vi "Set One Filter.vi"(8 "error in (no error)":errorcluster, 9 "Position (0:4)":i32, 10 "Filter Wheel (0:n-1)":i32, 11 "Filter Wheel in":refnum<class "Filter Wheel.lvclass">) -> (0 "error out":errorcluster, 1 "Target Counts":i32, 2 "Curr Pos":i32, 3 "Filter Wheel out":refnum<class "Filter Wheel.lvclass">, 4 "Message":string, 6 "No Move?":bool)   [LabVIEW 2024, in "Filter Wheel.lvclass"]
uses:
  Filter Wheel Object/Filter Wheel.lvclass
  Filter Wheel Object/Filter Wheel.lvclass/Filter Wheel.ctl
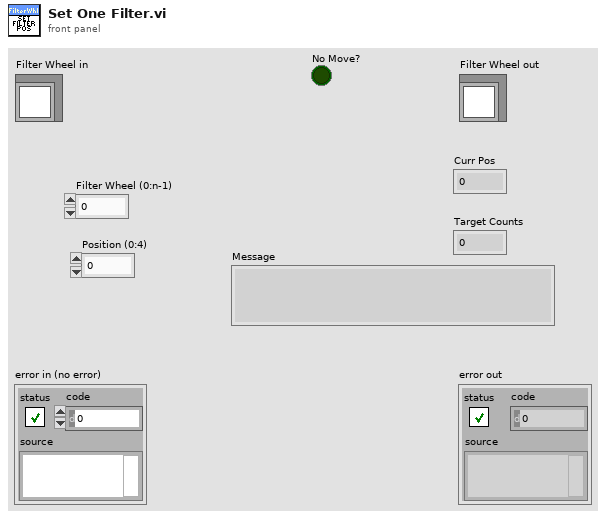
[diagram p1: front panel]
types:
  T1 = typedef "Filter Wheel Simulator.lvclass/Filter Wheel Move cluster.ctl" = cluster{"Wheel":i32, "Target Pos":i32}
  T2 = typedef "Filter Wheel.lvclass/Filter Wheel Details.ctl" = cluster{"Names":string[], "Relative Position":i32[], "Wheel Name":string, "Size":i32}
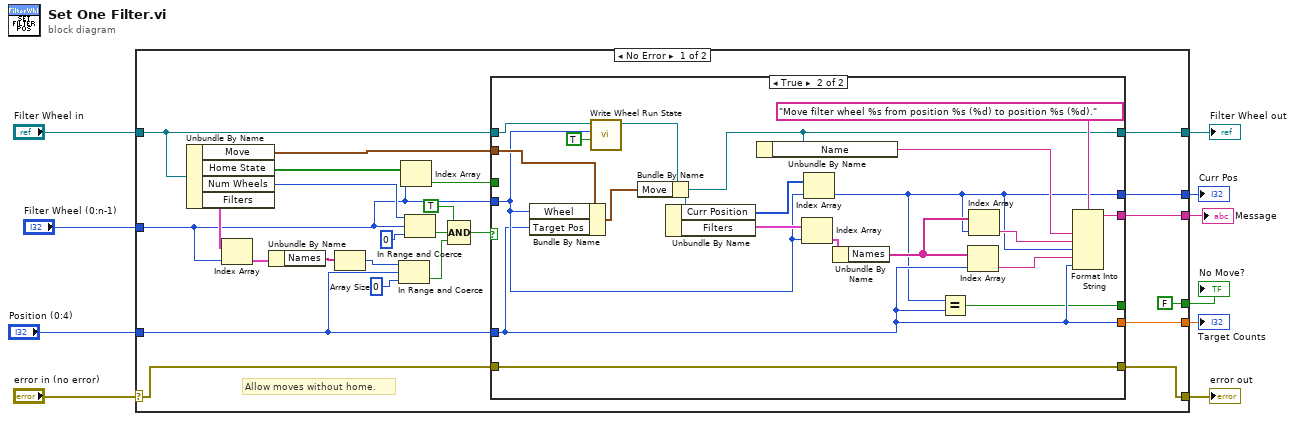
[diagram p0: block diagram]
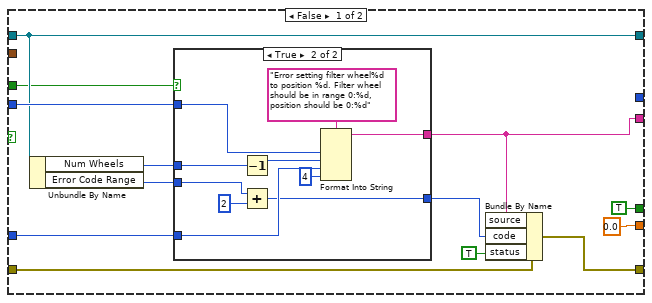
[diagram p2: hidden frame]
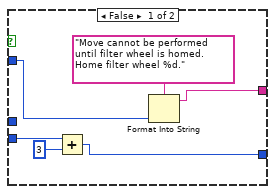
[diagram p3: hidden frame]
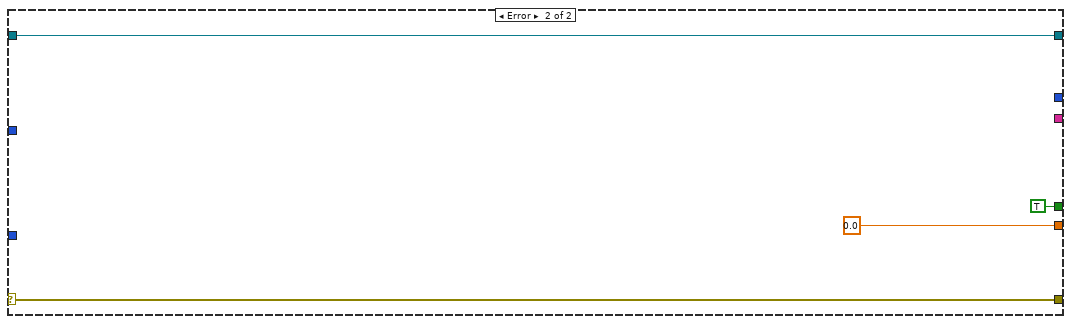
[diagram p4: hidden frame]
diagram:
  n1 = case shown="No Error" "error in (no error)" {
    selector: "error in (no error)" -> [w25 w87]
    tunnel: [w24 w87] -> w9
    tunnel: [w26 w86] -> w7
    tunnel: "Filter Wheel in" -> [w13 w86]
    tunnel: "Filter Wheel (0:n-1)" -> [w12 _]
    tunnel: "Position (0:4)" -> [w27 _]
    tunnel: [w19 0.0 ("Numeric")] -> w4
    tunnel: [w18 _] -> w3
    tunnel: [w17 _] -> w2
    tunnel: [FALSE TRUE] -> w1
    frame No Error {
      # "Allow moves without home."
      n2 = Unbundle By Name(w13) -> ("Move"=w28:T1, "Home State"=w16:bool[], "Num Wheels"=w33:i32, "Filters"=w23:T2[])
      n3 = Index Array(array=w23, index=w12) -> (element=w22:T2)
      n4 = Unbundle By Name(w22) -> ("Names"=w21:string[])
      n5 = Array Size(array=w21) -> (size(s)=w20:i32)
      n6 = In Range and Coerce(upper limit=w20, x=w27, lower limit=0) -> (In Range?=w30:bool)  [unwired: 1 out]
      n7 = Index Array(array=w16, index=w12) -> (element=w15:bool)
      n8 = In Range and Coerce(upper limit=w33, x=w12, lower limit=0) -> (In Range?=w31:bool)  [unwired: 1 out]
      n9 = Compound Arithmetic op=AND(TRUE ("value"), w31, w30) -> (w29:bool)
      n10 = case shown="True" w29 {
        tunnel: w28 -> [_ w82]
        tunnel: w12 -> [w47 w67]
        tunnel: w27 -> [w46 w66]
        tunnel: w13 -> [w45 w70]
        tunnel: [w45 w76] -> w26
        tunnel: w25 -> [w43 w83]
        tunnel: [w39 w83] -> w24
        tunnel: [0.0 ("Numeric") w66] -> w19
        tunnel: [_ w64] -> w18
        tunnel: [w37 w71] -> w17
        tunnel: w15 -> [w36 _]
        tunnel: [TRUE w65] -> _
        frame False {
          n11 = Unbundle By Name(w45) -> ("Num Wheels"=w44:i32, "Error Code Range"=w42:i32)
          n12 = case shown="True" w36 {
            tunnel: w47 -> [w52 w62]
            tunnel: w46 -> [_ w60]
            tunnel: w44 -> [_ w59]
            tunnel: w42 -> [w50 w57]
            tunnel: [w48 w55] -> w41
            tunnel: [w51 w54] -> w37
            frame False {
              n13 = Add(x=w50, y=3) -> (x+y=w48:i32)
              n14 = Format Into String(format string="Move cannot be performed until filter wheel is homed. Home filter wheel %d.", w52) -> (resulting string=w51:string)  [unwired: 2 in, 1 out]
            }
            frame True {
              n15 = Decrement(x=w59) -> (x-1=w58:i32)
              n16 = Add(x=w57, y=2) -> (x+y=w55:i32)
              n17 = Format Into String(format string="Error setting filter wheel%d to position %d. Filter wheel should be in range 0:%d, position should be 0:%d", w62, w58, w60, 4 ("input 4")) -> (resulting string=w54:string)  [unwired: 2 in, 1 out]
            }
          }
          n18 = Bundle By Name(cluster=w43, "source"=w37, "code"=w41, "status"=TRUE) -> (w39:errorcluster)
        }
        frame True {
          n19 = Bundle By Name(cluster=w82, "Wheel"=w67, "Target Pos"=w66) -> (w81:T1)
          n20 = call-dynamic "Write Wheel Run State.vi"("Run"=TRUE, "Wheel"=w67, "Filter Wheel in"=w70) -> ("Filter Wheel out"=w69:refnum<class "Filter Wheel.lvclass">)  [unwired: 7 in, 1 out]
          n21 = Bundle By Name(cluster=w69, "Move"=w81) -> (w76:refnum<class "Filter Wheel.lvclass">)
          n22 = Unbundle By Name(w76) -> ("Curr Position"=w79:i32[], "Filters"=w78:T2[])
          n23 = Unbundle By Name(w76) -> ("Name"=w75:string)
          n24 = Index Array(array=w78, index=w67) -> (element=w80:T2)
          n25 = Index Array(array=w79, index=w67) -> (element=w64:i32)
          n26 = Unbundle By Name(w80) -> ("Names"=w74:string[])
          n27 = Equal?(x=w64, y=w66) -> (x = y?=w65:bool)
          n28 = Index Array(array=w74, index=w66) -> (element=w72:string)
          n29 = Index Array(array=w74, index=w64) -> (element=w73:string)
          n30 = Format Into String(format string="Move filter wheel %s from position %s (%d) to position %s (%d).", w75, w73, w64, w72, w66) -> (resulting string=w71:string)  [unwired: 2 in, 1 out]
        }
      }
    }
    frame Error {
    }
  }
  "error out" <- w9
  "Filter Wheel out" <- w7
  "Target Counts" <- w4
  "Curr Pos" <- w3
  "Message" <- w2
  "No Move?" <- w1
